vi "Receive Message.vi"(8 "error in (no error)":errorcluster, 9 "timeout ms (-1)":i32=-1, 11 "TCP Stream in":refnum<class "TCP Stream.lvclass">) -> (0 "error out":errorcluster, 1 "Timed out?":bool, 2 "Message":refnum<class "Message.lvclass">, 3 "TCP Stream out":refnum<class "TCP Stream.lvclass">, 4 "priority":i32)   [LabVIEW 2020, in "TCP Stream.lvclass"]
uses:
  TCP Stream.lvclass
  Abstract Classes/Message Stream/Message Stream.lvclass
  Abstract Classes/Message Flattener/Message Flattener.lvclass
  Abstract Classes/Cipher/Cipher.lvclass
  <vilib>/ActorFramework/Message/Message.lvclass
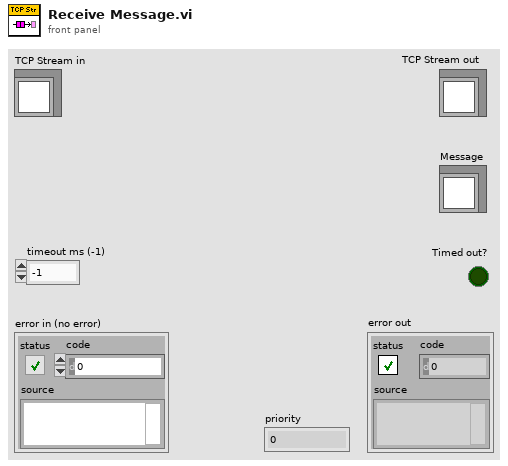
[diagram p1: front panel]
types:
  T1 = enum16{"Standard", "Buffered", "CRLF", "Immediate"}
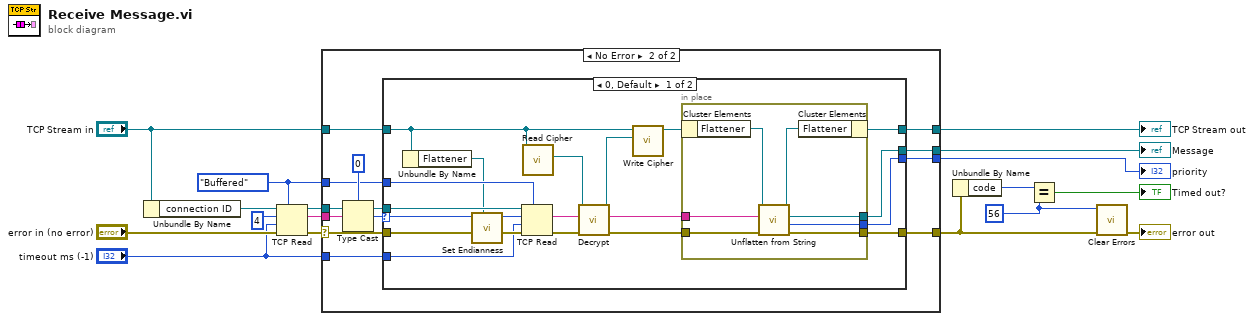
[diagram p0: block diagram]
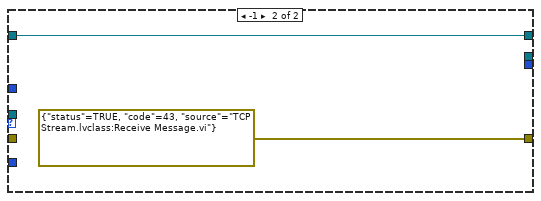
[diagram p3: hidden frame]
diagram:
  w1 = 56 ("x")
  w5 = T1."Buffered" ("mode (standard)")
  n1 = Unbundle By Name("TCP Stream in") -> ("connection ID"=w4:refnum<k5>)
  n2 = TCP Read(connection ID=w4, bytes to read=4, error in (no error)="error in (no error)", 7:w5, 9:"timeout ms (-1)") -> (connection ID out=w7:refnum<k5>, data out=w8:string, error out=w6:errorcluster)
  n3 = case shown="No Error" w6 {
    selector: w6 -> [w19 w28]
    tunnel: w8 -> [_ w31]
    tunnel: [w19 w25] -> w3
    tunnel: w7 -> [_ w29]
    tunnel: "timeout ms (-1)" -> [_ w27]
    tunnel: w5 -> [_ w26]
    tunnel: [_ w24] -> w11
    tunnel: [_ w23] -> w13
    tunnel: "TCP Stream in" -> [w18 w22]
    tunnel: [w18 w21] -> w15
    frame Error {
    }
    frame No Error {
      n4 = Type Cast(type=0 ("bytes to read"), x=w31) -> (*(type *) &x=w20:i32)
      n5 = case shown="0, Default" w20 {
        selector: w20 -> [w35 _]
        tunnel: w29 -> [w50 _]
        tunnel: w28 -> [w49 _]
        tunnel: w27 -> [w48 _]
        tunnel: w26 -> [w47 _]
        tunnel: [w40 errorcluster {"status"=TRUE, "code"=43, "source"="TCP Stream.lvclass:Receive Message.vi"} ("error out")] -> w25
        tunnel: [w39 _] -> w24
        tunnel: [w38 _] -> w23
        tunnel: w22 -> [w33 w58]
        tunnel: [w36 w58] -> w21
        frame 0, Default {
          n6 = Unbundle By Name(w33) -> ("Flattener"=w32:refnum<class "Message Flattener.lvclass">)
          n7 = call-dynamic "Set Endianness.vi"("Message Flattener in"=w32, "bytes to read"=w35) -> ("bytes to read"=w34:i32)  [unwired: 9 in]
          n8 = TCP Read(connection ID=w50, bytes to read=w34, error in (no error)=w49, 7:w47, 9:w48) -> (data out=w45:string, error out=w46:errorcluster)  [unwired: 1 out]
          n9 = call "Read Cipher.vi"("Message Stream in"=w33) -> ("Cipher.lvclass"=w44:refnum<class "Cipher.lvclass">)  [unwired: 10 in]
          n10 = call-dynamic "Decrypt.vi"("error in (no error)"=w46, "Ciphertext"=w45, "Cipher in"=w44) -> ("error out"=w42:errorcluster, "Plaintext"=w41:string, "Cipher out"=w43:refnum<class "Cipher.lvclass">)  [unwired: 6 in]
          n11 = call "Write Cipher.vi"("Cipher"=w43, "Message Stream in"=w33) -> ("Message Stream out"=w37:refnum<class "TCP Stream.lvclass">)  [unwired: 9 in]
          n12 = in-place {
            in-place-border: w42 -> [w57]
            in-place-border: w41 -> [w56]
            in-place-border: [w55] -> w40
            in-place-border: [w54] -> w39
            in-place-border: [w53] -> w38
            n13 = in-place-cluster #1(w37) -> ("Flattener"=w52:refnum<class "Message Flattener.lvclass">)
            n14 = call-dynamic "Unflatten from String.vi"("error in (no error)"=w57, "Flattened String"=w56, "Message Flattener in"=w52) -> ("error out"=w55:errorcluster, "priority"=w53:i32, "Message"=w54:refnum<class "Message.lvclass">, "Message Flattener out"=w51:refnum<class "Message Flattener.lvclass">)  [unwired: 5 in]
            n15 = in-place-cluster #1("Flattener"=w51) -> (w36:refnum<class "TCP Stream.lvclass">)
          }
        }
        frame -1 {
        }
      }
    }
  }
  "TCP Stream out" <- w15
  "Message" <- w11
  "priority" <- w13
  n16 = Unbundle By Name(w3) -> ("code"=w2:i32)
  n17 = Equal?(x=w2, y=w1) -> (x = y?=→"Timed out?":bool)
  n18 = call <vilib>:"Clear Errors.vi"("error in (no error)"=w3, "specific error code to clear (0: all)"=w1) -> ("error out"=→"error out":errorcluster)  [unwired: 4 in, 1 out]
